vi "locker-unlock.vi"(8 "error in (no error)":errorcluster, 11 "locker":refnum<queue>) -> (0 "error out":errorcluster, 3 "locker out":refnum<queue>)   [LabVIEW 2017]
doc: "Returns the locker so that a waiting locker-lock call can proceed."
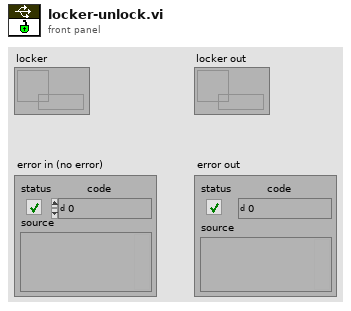
[diagram p1: front panel]
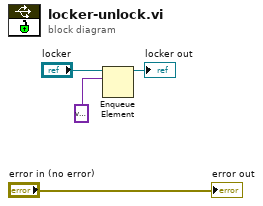
[diagram p0: block diagram]
diagram:
  n1 = Enqueue Element(queue="locker", element=variant) -> (queue out=→"locker out":refnum<queue>)  [unwired: 2 in, 2 out]
  "error out" <- "error in (no error)"
